vi "Write IsElite.vi"(8 "error in (no error)":errorcluster, 10 "IsElite":bool, 11 "IChromosome in":refnum<class "IChromosome.lvclass">) -> (0 "error out":errorcluster, 3 "IChromosome out":refnum<class "IChromosome.lvclass">)   [LabVIEW 2016, in "IChromosome.lvclass"]
uses:
  IChromosome.lvclass
  IChromosome.lvclass/IChromosome.ctl
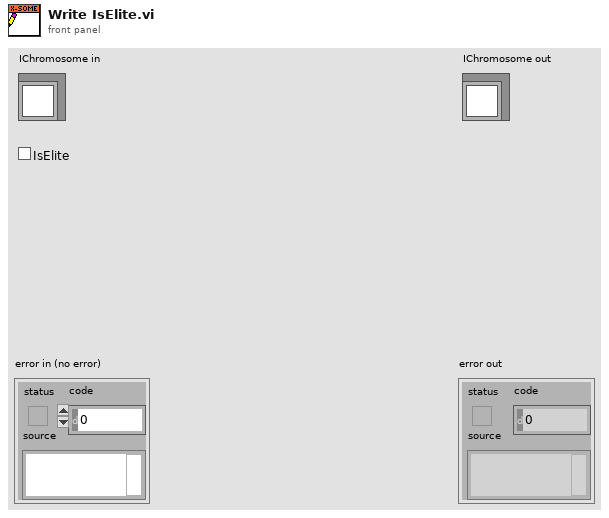
[diagram p1: front panel]
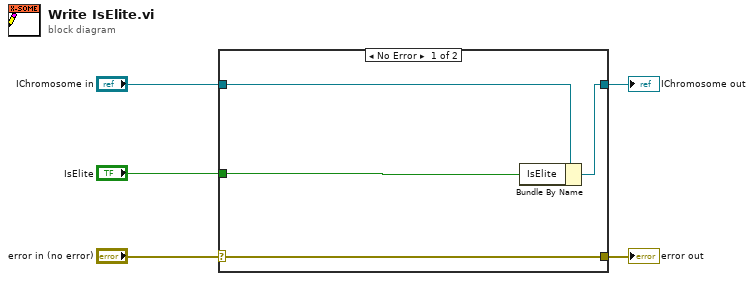
[diagram p0: block diagram]
diagram:
  n1 = case shown="No Error" "error in (no error)" {
    selector: "error in (no error)" -> [w9 w10]
    tunnel: [w9 w10] -> w4
    tunnel: [w7 w11] -> w2
    tunnel: "IChromosome in" -> [w8 w11]
    tunnel: "IsElite" -> [w6 _]
    frame No Error {
      n2 = Bundle By Name(cluster=w8, "IsElite"=w6) -> (w7:refnum<class "IChromosome.lvclass">)
    }
    frame Error {
    }
  }
  "error out" <- w4
  "IChromosome out" <- w2
